vi "Add to Bus (Collection).vi"(0 "reference fpga in":refnum<class "niUSRP Reference FPGA v1.lvclass">, 5 "subsystems":refnum<class "Address Space Collection.lvclass">) -> (4 "reference fpga out":refnum<class "niUSRP Reference FPGA v1.lvclass">)   [LabVIEW 2025, in "niUSRP Reference FPGA v1.lvclass"]
uses:
  niUSRP Reference FPGA v1.lvclass
  <instrlib>/_niInstr/Instruction Framework/v1/FPGA/Interfaces/Address Space Collection/Address Space Collection.lvclass
  niUSRP Reference FPGA v1.lvclass/niUSRP Reference FPGA v1.ctl
  <instrlib>/_niInstr/Instruction Framework/v1/FPGA/Top Level Bus/Register Configuration/Register Configuration.lvclass
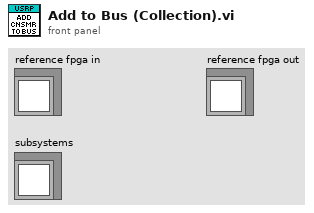
[diagram p1: front panel]
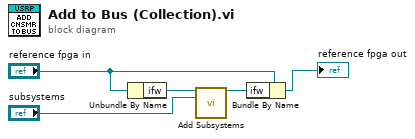
[diagram p0: block diagram]
diagram:
  n1 = Unbundle By Name("reference fpga in") -> ("ifw"=w2:refnum<class "Register Configuration.lvclass">)
  n2 = call-dynamic "Add Subsystems.vi"("register configuration in"=w2, "subsystems"="subsystems") -> ("register configuration out"=w3:refnum<class "Register Configuration.lvclass">)  [unwired: 13 in]
  n3 = Bundle By Name(cluster="reference fpga in", "ifw"=w3) -> (→"reference fpga out":refnum<class "niUSRP Reference FPGA v1.lvclass">)
